vi "TRITON_READ_TEMP_COMMAND.vi"(1 "Temperature Channel":i32) -> (0 "Command String":string)   [LabVIEW 2009]
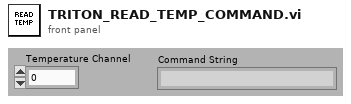
[diagram p1: front panel]
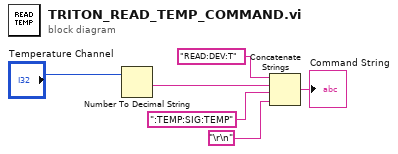
[diagram p0: block diagram]
diagram:
  n1 = Number To Decimal String(number="Temperature Channel") -> (decimal integer string=w4:string)  [unwired: 1 in]
  n2 = Concatenate Strings("READ:DEV:T", w4, ":TEMP:SIG:TEMP", "\r\n") -> (→"Command String":string)
